vi "pmu_Update Leap Second.vi"(9 "leap second direction":bool, 10 "leap seconds":i8, 11 "time stamp":timestamp) -> (1 "leap second status":T1, 2 "leap seconds out":i8, 3 "time stamp out":timestamp, 5 "status":enum16{"Unlocked", "Not Occurred", "Occurred"}(ring))   [LabVIEW 2015, in "NI_EP_PMU.lvlib"]
uses:
  <vilib>/addons/Electrical Power/PMU/NI_EP_PMU.lvlib
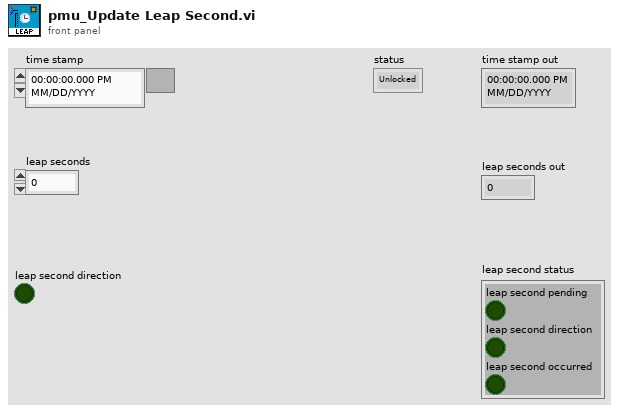
[diagram p1: front panel]
types:
  T1 = cluster{"leap second pending":bool, "leap second direction":bool, "leap second occurred":bool}
  T2 = enum16{"Not pending", "Pending", "Occurred", "Cleared"}
  T3 = typedef "LVDateTimeRec.ctl" = cluster{"fractional second":dbl, "second":i32, "minute":i32, "hour":i32, "day of month":i32, "month":i32, "year":i32, "day of week":i32, "day of year":i32, "DST":i32}
  T4 = cluster{bool, "leap second direction":bool, bool}
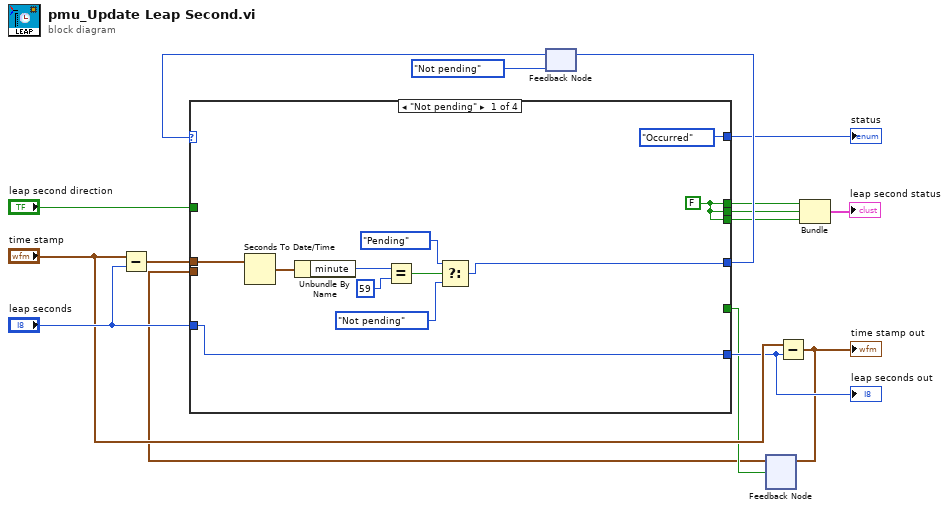
[diagram p0: block diagram]
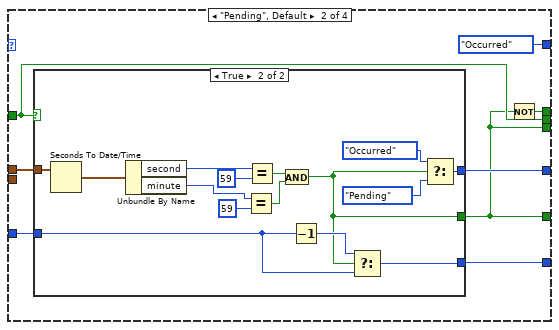
[diagram p2: hidden frame]
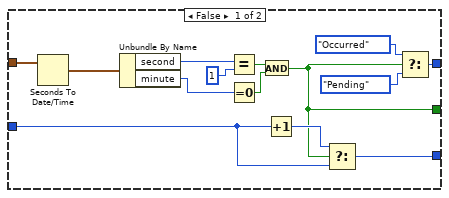
[diagram p3: hidden frame]
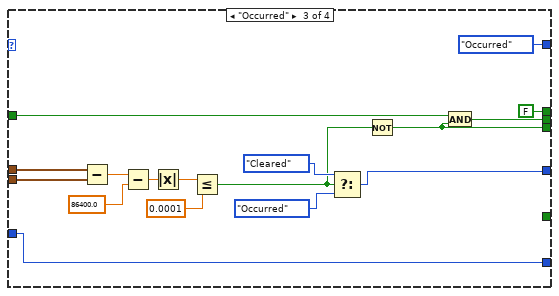
[diagram p4: hidden frame]
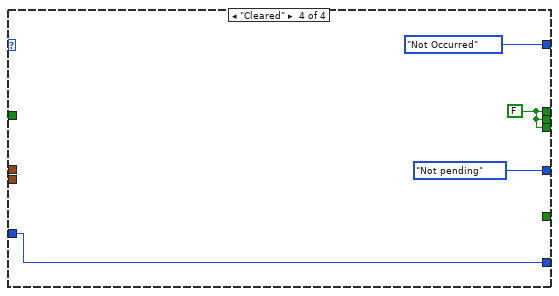
[diagram p5: hidden frame]
diagram:
  n1 = Subtract(x="time stamp", y="leap seconds") -> (x-y=w14:timestamp)
  n2 = feedback #1(T2."Not pending" ("f")) -> (w15:T2)
  n3 = feedback #2() -> (w6:timestamp)  [unwired: 1 in]
  n4 = case shown="\"Not pending\"" w15 {
    tunnel: w14 -> [w27 w35 w71 _]
    tunnel: "leap second direction" -> [_ w30 w73 _]
    tunnel: [w21 w34 w78 T2."Not pending" ("f")] -> w12
    tunnel: "leap seconds" -> [w19 w33 w75 w82]
    tunnel: [w19 w32 w75 w82] -> w9
    tunnel: [_ w28 _ _] -> w8
    tunnel: w6 -> [_ _ w81 _]
    tunnel: [enum16{"Unlocked", "Not Occurred", "Occurred"}."Occurred" ("f") enum16{"Unlocked", "Not Occurred", "Occurred"}."Occurred" ("f") enum16{"Unlocked", "Not Occurred", "Occurred"}."Occurred" ("f") enum16{"Unlocked", "Not Occurred", "Occurred"}."Not Occurred" ("f")] -> w5
    tunnel: [w18 w29 FALSE w83] -> w3
    tunnel: [w18 w30 w74 w83] -> w2
    tunnel: [w18 w28 w72 w83] -> w1
    frame "Not pending" {
      w18 = FALSE
      n5 = Seconds To Date/Time(time stamp (now)=w27) -> (date time rec=w26:T3)  [unwired: 1 in]
      n6 = Unbundle By Name(w26) -> ("minute"=w25:i32)
      n7 = Equal?(x=w25, y=59) -> (x = y?=w17:bool)
      n8 = Select(t=T2."Pending" ("f"), s=w17, f=T2."Not pending") -> (s? t:f=w21:T2)
    }
    frame "Pending", Default {
      n9 = case shown="True" w30 {
        tunnel: w35 -> [w49 w64]
        tunnel: [w47 w62] -> w34
        tunnel: w33 -> [w45 w60]
        tunnel: [w44 w59] -> w32
        tunnel: [w37 w51] -> w28
        frame False {
          n10 = Seconds To Date/Time(time stamp (now)=w49) -> (date time rec=w48:T3)  [unwired: 1 in]
          n11 = Unbundle By Name(w48) -> ("second"=w39:i32, "minute"=w38:i32)
          n12 = Equal?(x=w39, y=1) -> (x = y?=w41:bool)
          n13 = Equal To 0?(x=w38) -> (x = 0?=w36:bool)
          n14 = And(x=w41, y=w36) -> (x .and. y?=w37:bool)
          n15 = Increment(x=w45) -> (x+1=w46:i8)
          n16 = Select(t=w46, s=w37, f=w45) -> (s? t:f=w44:i8)
          n17 = Select(t=T2."Occurred" ("f"), s=w37, f=T2."Pending") -> (s? t:f=w47:T2)
        }
        frame True {
          n18 = Seconds To Date/Time(time stamp (now)=w64) -> (date time rec=w63:T3)  [unwired: 1 in]
          n19 = Unbundle By Name(w63) -> ("second"=w55:i32, "minute"=w52:i32)
          n20 = Equal?(x=w52, y=59) -> (x = y?=w50:bool)
          n21 = Equal?(x=w55, y=59) -> (x = y?=w56:bool)
          n22 = And(x=w56, y=w50) -> (x .and. y?=w51:bool)
          n23 = Decrement(x=w60) -> (x-1=w61:i8)
          n24 = Select(t=w61, s=w51, f=w60) -> (s? t:f=w59:i8)
          n25 = Select(t=T2."Occurred" ("f"), s=w51, f=T2."Pending") -> (s? t:f=w62:T2)
        }
      }
      n26 = Not(x=w28) -> (.not. x?=w29:bool)
    }
    frame "Occurred" {
      n27 = Subtract(x=w71, y=w81) -> (x-y=w70:dbl)
      n28 = Subtract(x=w70, y=86400.0) -> (x-y=w68:dbl)
      n29 = Absolute Value(x=w68) -> (abs(x)=w69:dbl)
      n30 = Less Or Equal?(x=w69, y=0.0001) -> (x <= y?=w65:bool)
      n31 = Select(t=T2."Cleared" ("f"), s=w65, f=T2."Occurred") -> (s? t:f=w78:T2)
      n32 = Not(x=w65) -> (.not. x?=w72:bool)
      n33 = And(x=w73, y=w72) -> (x .and. y?=w74:bool)
    }
    frame "Cleared" {
      w83 = FALSE
    }
  }
  "leap seconds out" <- w9
  "status" <- w5
  n34 = feedback-in #1(w12) -> ()
  n35 = Subtract(x="time stamp", y=w9) -> (x-y=w7:timestamp)
  "time stamp out" <- w7
  n36 = feedback-in #2(w7, w8) -> ()
  n37 = Bundle(w3, "leap second direction"=w2, w1) -> (→"leap second status":T4)  [unwired: 1 in]
